vi "Constructor with Reference Fit.vi"(10 "Direction":bool, 11 "Reference Fit":refnum<class "Sinusoidal Fit.lvclass">) -> (3 "Halfwave Sinusoidal Fit out":refnum<class "Halfwave Sinusoidal Fit.lvclass">)   [LabVIEW 2016, in "Halfwave Sinusoidal Fit.lvclass"]
uses:
  Halfwave Sinusoidal Fit.lvclass
  Sinusoidal Fit.lvclass
  Halfwave Sinusoidal Fit.lvclass/Halfwave Sinusoidal Fit.ctl
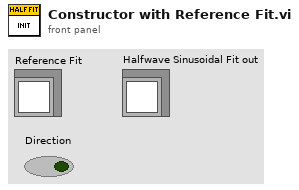
[diagram p1: front panel]
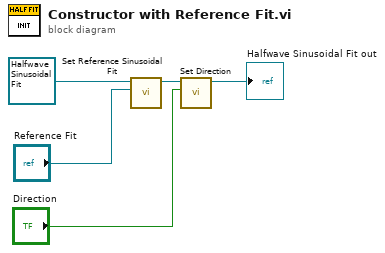
[diagram p0: block diagram]
diagram:
  n1 = call "Set Reference Sinusoidal Fit.vi"("Sinusoidal Fit.lvclass"="Reference Fit", "Halfwave Sinusoidal Fit in"=refnum<class "Halfwave Sinusoidal Fit.lvclass"> refnum ("Halfwave Sinusoidal Fit.lvclass")) -> ("Halfwave Sinusoidal Fit out"=w3:refnum<class "Halfwave Sinusoidal Fit.lvclass">)  [unwired: 8 in, 1 out]
  n2 = call-dynamic "Set Direction.vi"("Direction"="Direction", "Halfwave Sinusoidal Fit in"=w3) -> ("Halfwave Sinusoidal Fit out"=→"Halfwave Sinusoidal Fit out":refnum<class "Halfwave Sinusoidal Fit.lvclass">)  [unwired: 8 in, 1 out]
